vi "Indicador lamina.vi"() -> ()   [LabVIEW 2018]
panel:
  in  "Numeric Control":dbl
  in  "Boolean":bool
  out "Dial":u8(knob) max=16 step=1 scale=0.0..16.0
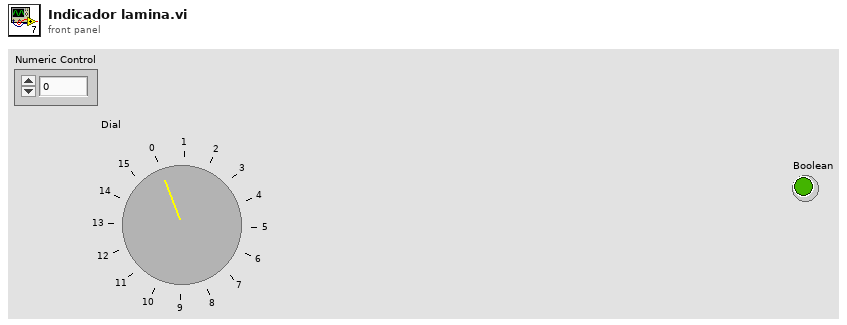
[diagram p1: front panel]
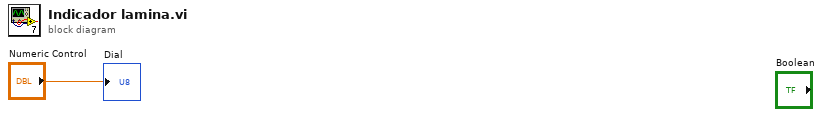
[diagram p0: block diagram]
diagram:
  "Dial" <- "Numeric Control"
